vi "String to Config.vi"(8 "error in (no error)":errorcluster, 10 "string input":string, 11 "DSF Configuration Reference in":T1) -> (0 "error out":errorcluster, 3 "DSF Configuration Reference out":T1)   [LabVIEW 2017, in "DSF Configuration API.lvlib"]
uses:
  DSF Configuration API.lvlib
  Controls/Session/DSF Configuration Reference.ctl
  Controls/Session/Config Data.ctl
  Controls/DSF File Format/DSF Config.ctl
  Public/Controls/Version Info.ctl
  Controls/DSF File Format/DSF Plugin.ctl
  Public/Controls/DSF Plugin Info.ctl
  Public/Controls/DSF Timing Info.ctl
  Controls/DSF File Format/DSF Group.ctl
  Public/Controls/DSF Group Info.ctl
  Controls/DSF File Format/DSF Transfer.ctl
  Public/Controls/DSF Transfer Info.ctl
  Controls/DSF File Format/DSF Channel.ctl
  Public/Controls/DSF Channel Info.ctl
  Controls/DSF File Format/DSF Settings.ctl
  Public/Controls/DSF Settings Info.ctl
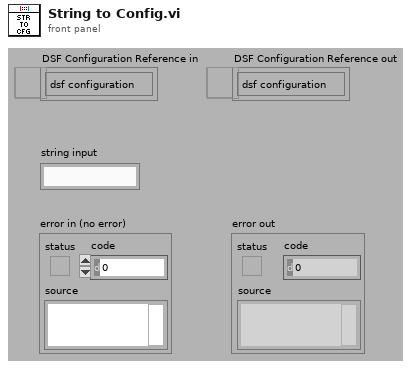
[diagram p1: front panel]
types:
  T1 = typedef "DSF Configuration API.lvlib/DSF Configuration Reference.ctl" = refnum<data-value>
  T2 = typedef "DSF Configuration API.lvlib/DSF Config.ctl" = cluster{"dsfversion":T3, "version":T3, "plugins":T4[], "groups":T7[], "transfers":T9[], "channels":T11[], "settings":T13[]}
  T3 = typedef "DSF Configuration API.lvlib/Version Info.ctl" = cluster{"major":u32, "minor":u32, "fix":u32, "build":string}
  T4 = typedef "DSF Configuration API.lvlib/DSF Plugin.ctl" = cluster{"id":string, "values":T5}
  T5 = typedef "DSF Configuration API.lvlib/DSF Plugin Info.ctl" = cluster{"type":string, "timing":T6, "group ids":string[], "settings id":string}
  T6 = typedef "DSF Configuration API.lvlib/DSF Timing Info.ctl" = cluster{"priority":i32, "decimation":i32, "offset":i32}
  T7 = typedef "DSF Configuration API.lvlib/DSF Group.ctl" = cluster{"id":string, "values":T8}
  T8 = typedef "DSF Configuration API.lvlib/DSF Group Info.ctl" = cluster{"direction":i32, "timing":T6, "transfer ids":string[], "settings id":string}
  T9 = typedef "DSF Configuration API.lvlib/DSF Transfer.ctl" = cluster{"id":string, "values":T10}
  T10 = typedef "DSF Configuration API.lvlib/DSF Transfer Info.ctl" = cluster{"byte order":i32, "channel ids":string[], "settings id":string}
  T11 = typedef "DSF Configuration API.lvlib/DSF Channel.ctl" = cluster{"id":string, "values":T12}
  T12 = typedef "DSF Configuration API.lvlib/DSF Channel Info.ctl" = cluster{"count":i32, "offset":i32, "data type":i32, "resource path":string, "settings id":string}
  T13 = typedef "DSF Configuration API.lvlib/DSF Settings.ctl" = cluster{"id":string, "values":T14}
  T14 = typedef "DSF Configuration API.lvlib/DSF Settings Info.ctl" = cluster{"key":string, "value":string}[]
  T15 = typedef "DSF Configuration API.lvlib/Config Data.ctl" = cluster{"dsf configuration":T2, "path":path, "dirty":bool}
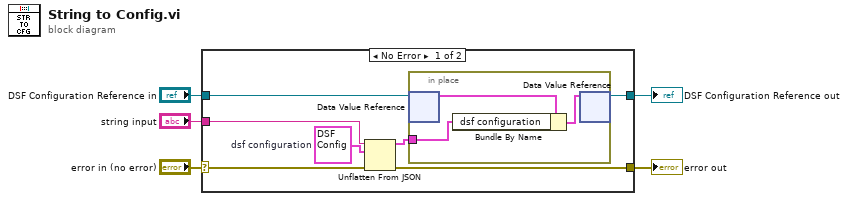
[diagram p0: block diagram]
diagram:
  n1 = case shown="No Error" "error in (no error)" {
    selector: "error in (no error)" -> [w9 w17]
    tunnel: "DSF Configuration Reference in" -> [w7 w16]
    tunnel: [w6 w16] -> w2
    tunnel: "string input" -> [w10 _]
    tunnel: [w12 w17] -> w4
    frame No Error {
      w11 = T2 {"dsfversion"={"major"=0, "minor"=0, "fix"=0, "build"=""}, "version"={"major"=0, "minor"=0, "fix"=0, "build"=""}, "plugins"=[], "groups"=[], "transfers"=[], "channels"=[], "settings"=[]}  # dsf configuration
      n2 = Unflatten From JSON(JSON string=w10, type and defaults=w11, error in (no error)=w9) -> (value=w8:T2, error out=w12:errorcluster)  [unwired: 4 in]
      n3 = in-place {
        in-place-border: w8 -> [w15]
        n4 = in-place-dvr #1(w7) -> (w14:T15)  [unwired: 1 out]
        n5 = Bundle By Name(cluster=w14, "dsf configuration"=w15) -> (w13:T15)
        n6 = in-place-dvr #1(w13) -> (w6:T1)  [unwired: 1 out]
      }
    }
    frame Error {
    }
  }
  "error out" <- w4
  "DSF Configuration Reference out" <- w2
